vi "Get State.vi"(7 "Channel (1: Chan A)":i32(ring)=1 items=["System (To)", "Channel A", "Channel B", "Channel C", "Channel D", "Channel E", "Channel F", "Channel G", "Channel H"], 8 "error in (no error)":errorcluster, 11 "VISA resource name":refnum<visa-resource-name>) -> (0 "error out":errorcluster, 2 "State":bool, 3 "VISA resource name out":refnum<visa-resource-name>)   [LabVIEW 2012, in "Quantum Composers 9000 Series.lvlib"]
doc: "This VI is used to read the state of the selected channel or system timer (To)."
uses:
  Quantum Composers 9000 Series.lvlib
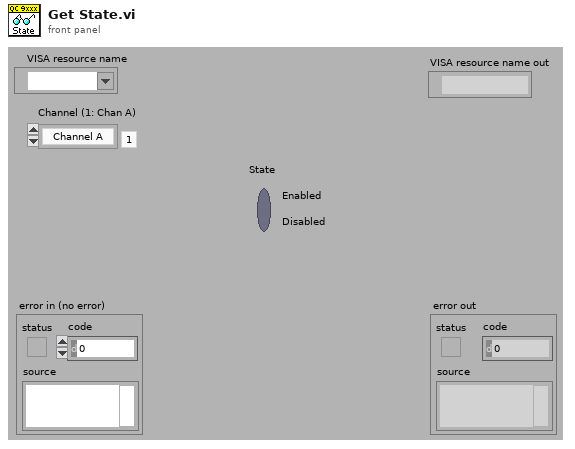
[diagram p1: front panel]
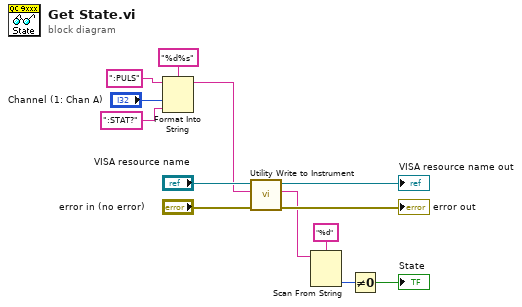
[diagram p0: block diagram]
diagram:
  n1 = Format Into String(format string="%d%s", initial string=":PULS", "Channel (1: Chan A)", ":STAT?") -> (resulting string=w2:string)  [unwired: 1 in, 1 out]
  n2 = call "Utility Write to Instrument.vi"("error in (no error)"="error in (no error)", "Write Buffer"=w2, "VISA resource name"="VISA resource name") -> ("error out"=→"error out":errorcluster, "Read Buffer"=w6:string, "VISA resource name out"=→"VISA resource name out":refnum<visa-resource-name>)  [unwired: 6 in]
  n3 = Scan From String(format string="%d", input string=w6) -> (output 1=w4:i32)  [unwired: 3 in, 3 out]
  n4 = Not Equal To 0?(x=w4) -> (x != 0?=→"State":bool)
